vi "scrollbar_min_max-point.vi"(7 "flipped":bool, 8 "error in (no error)":errorcluster, 10 "data_visible":i32, 11 "data_total":i32=-1) -> (0 "error out":errorcluster, 4 "scrollbar_doc_max":dbl, 6 "scrollbar_doc_min":dbl)   [LabVIEW 2015, in "lv-graph.lvlib"]
doc: "This VI can be used to determine the min/max values for the scrollbars to represent a given data set."
uses:
  lv-graph.lvlib
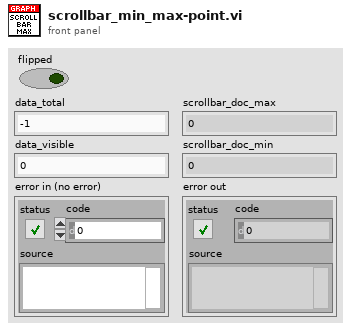
[diagram p1: front panel]
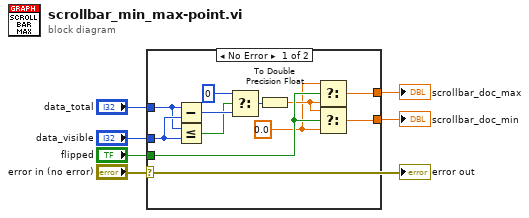
[diagram p0: block diagram]
diagram:
  n1 = case shown="No Error" "error in (no error)" {
    tunnel: "data_total" -> [w7 _]
    tunnel: "data_visible" -> [w17 _]
    tunnel: "flipped" -> [w12 _]
    tunnel: [w11 _] -> w3
    tunnel: [w10 _] -> w2
    frame No Error {
      w8 = 0.0 ("Scrollbar DocMin")
      n2 = Subtract(x=w7, y=w17) -> (x-y=w16:i32)
      n3 = Less Or Equal?(x=w7, y=w17) -> (x <= y?=w13:bool)
      n4 = Select(t=0, s=w13, f=w16) -> (s? t:f=w14:i32)
      n5 = To Double Precision Float(number=w14) -> (double precision float=w9:dbl)
      n6 = Select(t=w8, s=w12, f=w9) -> (s? t:f=w11:dbl)
      n7 = Select(t=w9, s=w12, f=w8) -> (s? t:f=w10:dbl)
    }
    frame Error {
    }
  }
  "scrollbar_doc_max" <- w3
  "scrollbar_doc_min" <- w2
  "error out" <- "error in (no error)"
